vi "Set Panel Color.vi"(3 "error in":errorcluster, 4 "Call Level (2)":i32=2, 5 "Panel Color (Gray)":u32(colorbox)=14869218) -> (0 "error out":errorcluster)   [LabVIEW 2010]
doc: "Set the LabView panel color."
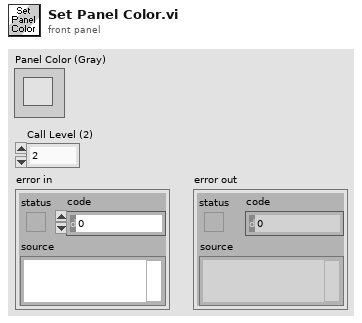
[diagram p1: front panel]
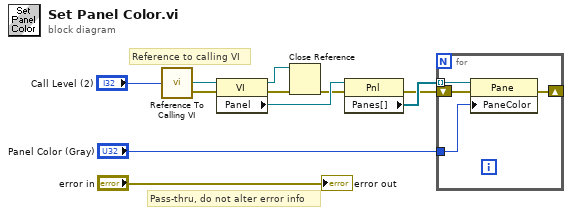
[diagram p0: block diagram]
diagram:
  # "Pass-thru, do not alter error info"
  # "Reference to calling VI"
  n1 = call "Reference To Calling VI.vi"("Call Level (2)"="Call Level (2)") -> ("error out"=w2:errorcluster, "VI Reference"=w3:refnum<vi>)  [unwired: 2 in]
  n2 = property class="VI"(reference=w3, error in=w2) -> (reference out=w10:refnum<vi>, error out=w11:errorcluster, "Panel"=w9:refnum<vi>)
  n3 = Close Reference(reference=w10, error in (no error)=w11) -> (error out=w7:errorcluster)
  n4 = property class="Pnl"(reference=w9, error in=w7) -> (error out=w6:errorcluster, "Panes[]"=w8:refnum<vi>[])  [unwired: 1 out]
  n5 = for {
    tunnel: w8 -> [w15] mode=indexing
    shift-right: [w13] -> _
    shift-left: w6 -> [w14]
    tunnel: "Panel Color (Gray)" -> [w12]
    n6 = property class="Pane"(reference=w15, error in=w14, "PaneColor"=w12) -> (error out=w13:errorcluster)  [unwired: 1 out]
  }
  "error out" <- "error in"
